vi "WaitPassRole_Init.vi"(0 "object in":refnum<class "WaitPassRole.lvclass">, 5 "error in (no error)":errorcluster) -> (14 "object out":refnum<class "WaitPassRole.lvclass">, 19 "error out":errorcluster)   [LabVIEW 2024, in "WaitPassRole.lvclass"]
uses:
  WaitPassRole.lvclass
  C:/Users/moise/Documents/GitHub/SSL_AI/Role_class/Role.lvclass
  Role_class/Role.lvclass
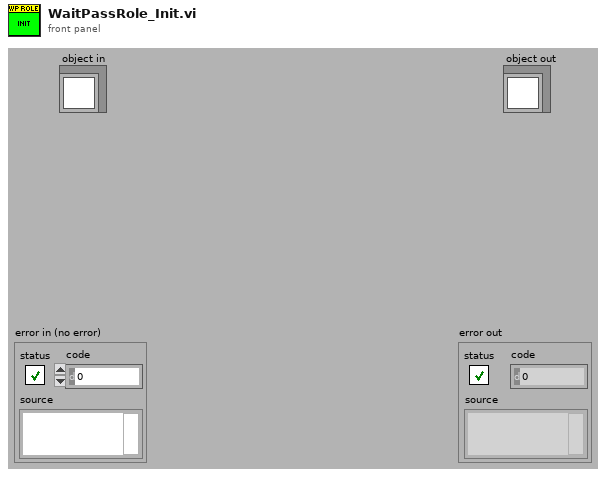
[diagram p1: front panel]
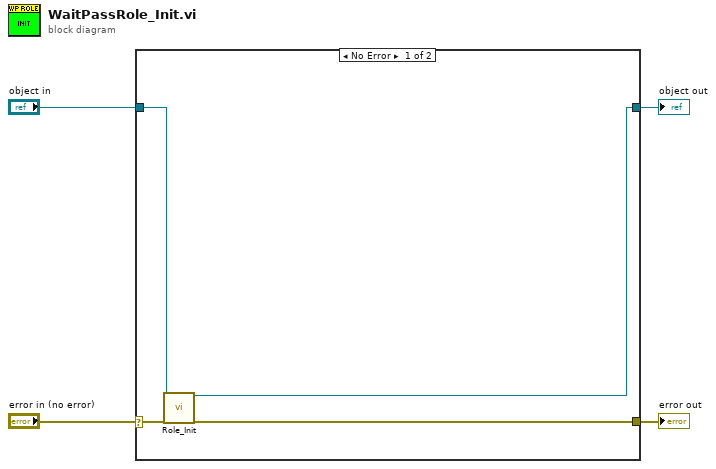
[diagram p0: block diagram]
diagram:
  n1 = case shown="No Error" "error in (no error)" {
    selector: "error in (no error)" -> [w8 w9]
    tunnel: [w5 w10] -> w4
    tunnel: "object in" -> [w6 w10]
    tunnel: [w7 w9] -> w1
    frame No Error {
      n2 = call "Role_Init.vi"("object in"=w6, "error in (no error)"=w8) -> ("object out"=w5:refnum<class "WaitPassRole.lvclass">, "error out"=w7:errorcluster)  [unwired: 16 in]
    }
    frame Error {
    }
  }
  "object out" <- w4
  "error out" <- w1
